vi "Write Configuration.lvlib_Configuration.lvclass.vi"(8 "error in (no error)":errorcluster, 10 "Hardware.lvlib:HW Configuration.lvclass":refnum<class "HW Configuration.lvclass">, 11 "CompactDAQ in":refnum<class "CompactDAQ.lvclass">) -> (0 "error out":errorcluster, 3 "CompactDAQ out":refnum<class "CompactDAQ.lvclass">)   [LabVIEW 2017, in "CompactDAQ.lvclass"]
uses:
  CompactDAQ.lvclass
  \\Mac\Home/Documents/MAL-Framework/user.lib/Common Components/Hardware/Hardware.lvclass
  <userlib>/Common Components/Hardware/HW Config/HW Configuration.lvclass
  CompactDAQ Configuration.lvclass
  CompactDAQ Configuration.lvclass/CompactDAQ Configuration.ctl
  <userlib>/Common Components/Hardware/Hardware.lvclass/Hardware.ctl
  <userlib>/Common Components/Hardware/DAQ/DAQ .lvclass
  <userlib>/Common Components/Hardware/Hardware.lvclass
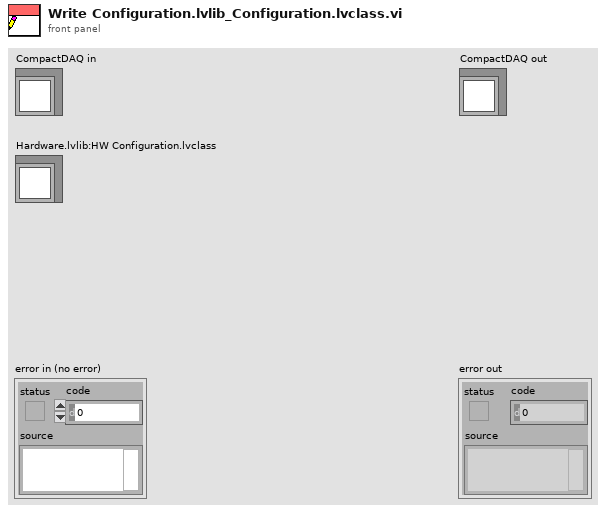
[diagram p1: front panel]
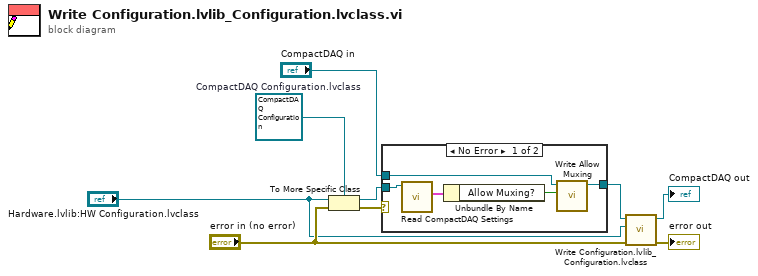
[diagram p0: block diagram]
diagram:
  w7 = refnum<class "CompactDAQ Configuration.lvclass"> refnum  # CompactDAQ Configuration.lvclass
  n1 = To More Specific Class(target class=w7, reference="Hardware.lvlib:HW Configuration.lvclass", error in="error in (no error)") -> (specific class reference=w2:refnum<class "CompactDAQ Configuration.lvclass">, error out=w5:errorcluster)
  n2 = case shown="No Error" w5 {
    tunnel: "CompactDAQ in" -> [w14 w15]
    tunnel: [w13 w15] -> w3
    tunnel: w2 -> [w12 _]
    frame No Error {
      n3 = call "Read CompactDAQ Settings.vi"("CompactDAQ Configuration in"=w12) -> ("CompactDAQ Settings"=w11:cluster{"Allow Muxing?":bool})  [unwired: 8 in, 2 out]
      n4 = Unbundle By Name(w11) -> ("Allow Muxing?"=w10:bool)
      n5 = call <userlib>:"Write Allow Muxing.vi"("Allow Muxing"=w10, "Hardware in"=w14) -> ("Hardware out"=w13:refnum<class "CompactDAQ.lvclass">)  [unwired: 8 in, 1 out]
    }
    frame Error {
    }
  }
  n6 = call-parent "Write Configuration.lvlib_Configuration.lvclass.vi"("error in (no error)"="error in (no error)", "Hardware.lvlib:HW Configuration.lvclass"="Hardware.lvlib:HW Configuration.lvclass", "Hardware in"=w3) -> ("error out"=→"error out":errorcluster, "Hardware out"=→"CompactDAQ out":refnum<class "CompactDAQ.lvclass">)  [unwired: 7 in]
